vi "TF_MotorCurrentOutput.vi"(1 "Motor Current Setpoint [A]":dbl) -> (0 "Motor Current Setpoint [V]":dbl)   [LabVIEW 2019]
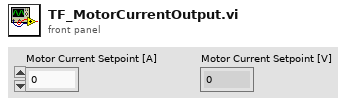
[diagram p1: front panel]
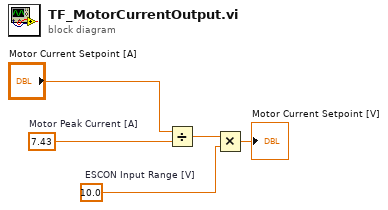
[diagram p0: block diagram]
diagram:
  w5 = 10.0  # ESCON Input Range [V]
  w3 = 7.43  # Motor Peak Current [A]
  n1 = Divide(x="Motor Current Setpoint [A]", y=w3) -> (x/y=w4:dbl)
  n2 = Multiply(x=w4, y=w5) -> (x*y=→"Motor Current Setpoint [V]":dbl)
